vi "kinectRead [DepthFrame].vi"(8 "Error In":errorcluster, 9 "Timeout (ms)":i32=5000, 11 "KinectSensor References in":T1) -> (0 "Error Out":errorcluster, 2 "frameData":dbl[](array[numeric]), 3 "KinectSensor References out":T1)   [LabVIEW 2011, in "LVH-KinectOne.lvlib"]
doc: "The data for this frame is stored as 16-bit unsigned integers, where each value represents the distance in millimeters. The maximum depth distance is 8 meters, although reliability starts to degrade at around 4.5 meters. Developers can use the depth frame to build custom tracking algorithms in cases where the BodyFrame isn’t enough."
uses:
  LVH-KinectOne.lvlib
  Type Defs/KinectSensor References.ctl
  Microsoft.Kinect
  C:/github/makerhub/KinectOne/LabVIEW/vi.lib/MakerHub/KinectOne/Private/Libs/BodyFrameDataInterface.dll
  Libs/BodyFrameDataInterface.dll
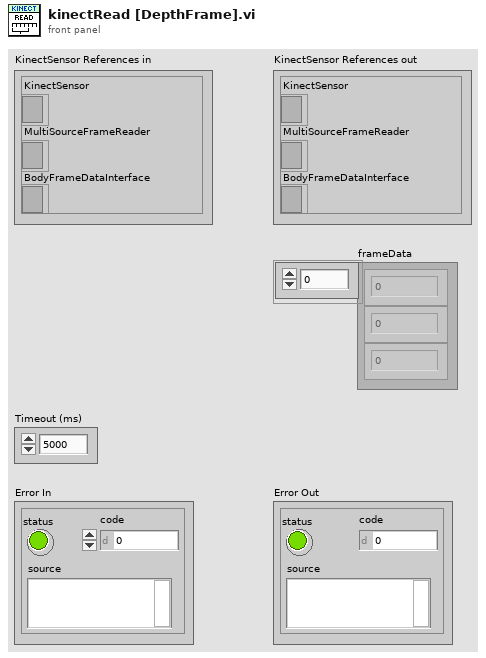
[diagram p1: front panel]
types:
  T1 = typedef "LVH-KinectOne.lvlib/KinectSensor References.ctl" = cluster{"KinectSensor":refnum<k24>, "MultiSourceFrameReader":refnum<k24>, "BodyFrameDataInterface":refnum<k24>}
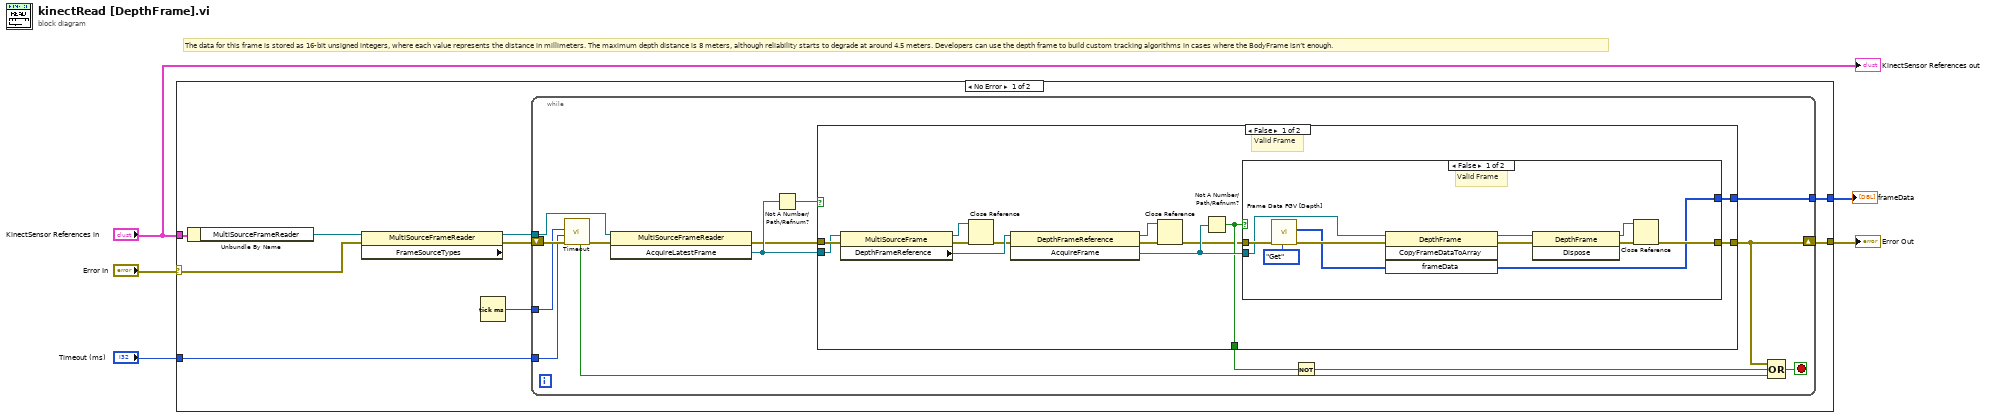
[diagram p0: block diagram]
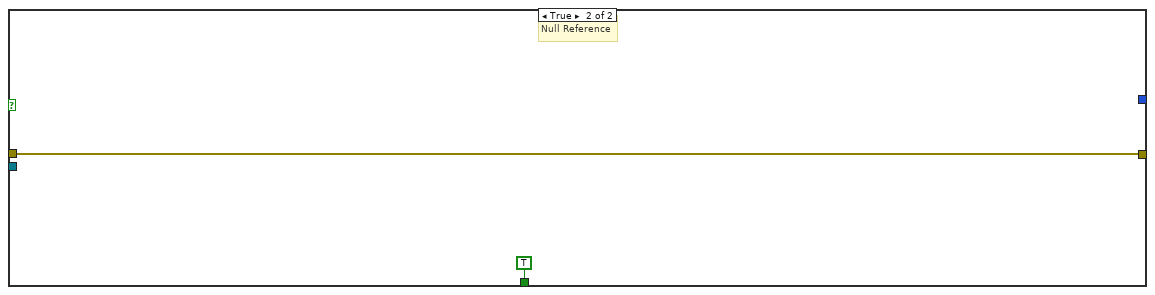
[diagram p3: hidden frame]
diagram:
  # "The data for this frame is stored as 16-bit unsigned integers, where each value represents the distance in millimeters. The maximum depth distance is 8 meters, although reliability starts to degrade at around 4.5 meters. Developers can use the depth frame to build custom tracking algorithms in cases where the BodyFrame isn’t enough."
  n1 = case shown="No Error" "Error In" {
    selector: "Error In" -> [w6 w56]
    tunnel: "KinectSensor References in" -> [w11 _]
    tunnel: [w10 w56] -> w4
    tunnel: [w9 _] -> w3
    tunnel: "Timeout (ms)" -> [w7 _]
    frame No Error {
      n2 = Unbundle By Name(w11) -> ("MultiSourceFrameReader"=w12:refnum<k24>)
      n3 = property class="MultiSourceFrameReader" props=["FrameSourceTypes"](reference=w12, error in=w6) -> (reference out=w14:refnum<k24>, error out=w13:errorcluster)  [unwired: 1 out]
      n4 = Tick Count (ms)() -> (millisecond timer value=w8:u32)
      n5 = while {
        tunnel: w14 -> [w24]
        shift-right: [w19] -> w10
        shift-left: w13 -> [w23]
        tunnel: [w25] -> w9
        tunnel: w8 -> [w21]
        tunnel: w7 -> [w20]
        stop <- w18 stop-if-true
        n6 = call "Timeout.vi"("error in (no error)"=w23, "Timeout (ms)"=w20, "Start Time"=w21) -> ("error out"=w22:errorcluster, "Timeout?"=w15:bool)  [unwired: 7 in]
        n7 = invoke class="MultiSourceFrameReader" method="AcquireLatestFrame"(reference=w24, error in=w22) -> (error out=w27:errorcluster, "AcquireLatestFrame"=w28:refnum<k24>)  [unwired: 1 in, 1 out]
        n8 = Not A Number/Path/Refnum?(number/path/refnum=w28) -> (NaN/Path/Refnum?=w26:bool)
        n9 = case shown="False" w26 {
          tunnel: w27 -> [w40 w54]
          tunnel: w28 -> [w37 _]
          tunnel: [w39 w54] -> w19
          tunnel: [w38 TRUE] -> w17
          tunnel: [w35 _] -> w25
          frame False {
            # "Valid Frame"
            n10 = property class="MultiSourceFrame"(reference=w37, error in=w40) -> (reference out=w33:refnum<k24>, error out=w34:errorcluster, "DepthFrameReference"=w36:refnum<k24>)
            n11 = Close Reference(reference=w33, error in (no error)=w34) -> (error out=w32:errorcluster)
            n12 = invoke class="DepthFrameReference" method="AcquireFrame"(reference=w36, error in=w32) -> (reference out=w30:refnum<k24>, error out=w31:errorcluster, "AcquireFrame"=w41:refnum<k24>)  [unwired: 1 in]
            n13 = Close Reference(reference=w30, error in (no error)=w31) -> (error out=w29:errorcluster)
            n14 = Not A Number/Path/Refnum?(number/path/refnum=w41) -> (NaN/Path/Refnum?=w38:bool)
            n15 = case shown="False" w38 {
              tunnel: w29 -> [w45 w53]
              tunnel: w41 -> [w44 _]
              tunnel: [w43 w53] -> w39
              tunnel: [w42 _] -> w35
              frame False {
                # "Valid Frame"
                n16 = call "Frame Data FGV [Depth].vi"("Command"=enum16{"Get", "Initialize"}."Get", "error in (no error)"=w45) -> ("error out"=w52:errorcluster, "Array"=w47:u16[])  [unwired: 8 in]
                n17 = invoke class="DepthFrame" method="CopyFrameDataToArray"(reference=w44, error in=w52, "frameData"=w47) -> (reference out=w48:refnum<k24>, error out=w49:errorcluster, "frameData"=w42:u16[])  [unwired: 1 in, 1 out]
                n18 = invoke class="DepthFrame" method="Dispose"(reference=w48, error in=w49) -> (reference out=w51:refnum<k24>, error out=w50:errorcluster)  [unwired: 1 in, 1 out]
                n19 = Close Reference(reference=w51, error in (no error)=w50) -> (error out=w43:errorcluster)
              }
              frame True {
                # "Null Reference"
              }
            }
          }
          frame True {
            # "Null Reference"
          }
        }
        n20 = Not(x=w17) -> (.not. x?=w16:bool)
        n21 = Compound Arithmetic op=OR(w19, w16, w15) -> (w18:bool)
      }
    }
    frame Error {
    }
  }
  "Error Out" <- w4
  "frameData" <- w3
  "KinectSensor References out" <- "KinectSensor References in"
